vi "Prog11.vi"() -> ()   [LabVIEW 2021]
panel:
  out "length 7":i32
  out "length 6":i32
  out "length 5":i32
  out "length 3":i32
  out "length 2":i32
  out "length":i32
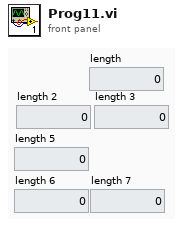
[diagram p1: front panel]
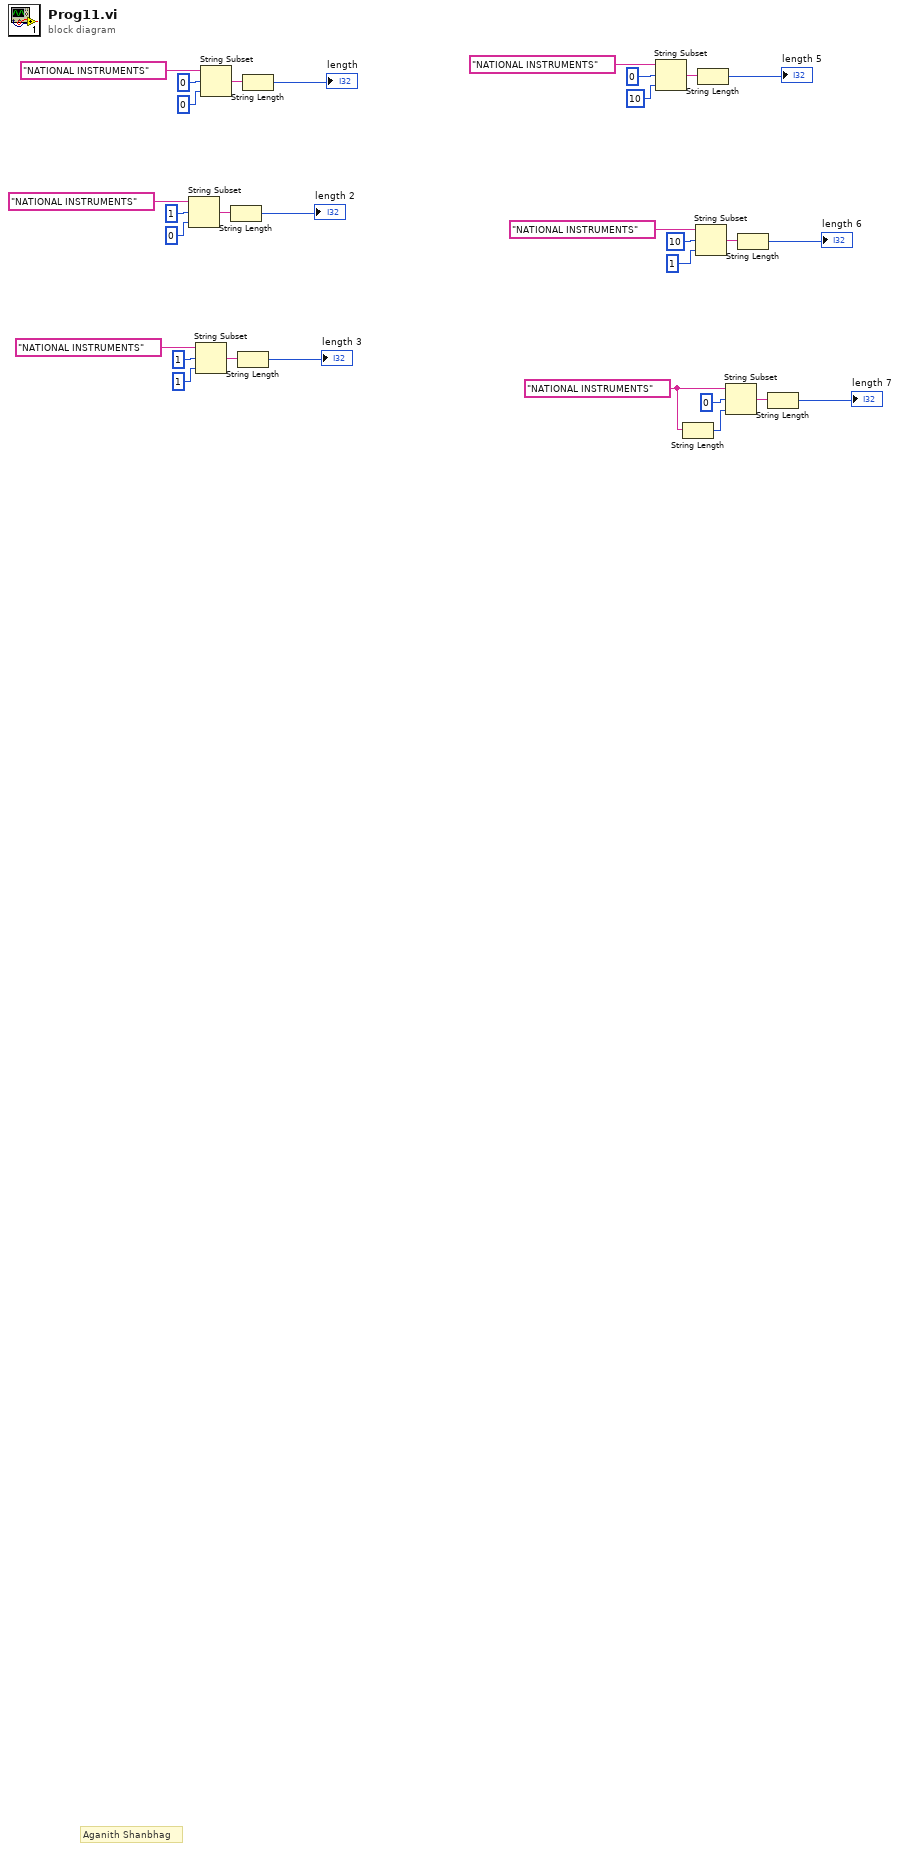
[diagram p0: block diagram]
diagram:
  w10 = "NATIONAL INSTRUMENTS"
  # "Aganith Shanbhag"
  n1 = String Subset(string="NATIONAL INSTRUMENTS", offset (0)=1, length (rest)=0 ("length (rest)")) -> (substring=w21:string)
  n2 = String Subset(string="NATIONAL INSTRUMENTS", offset (0)=1, length (rest)=1 ("length (rest)")) -> (substring=w8:string)
  n3 = String Subset(string="NATIONAL INSTRUMENTS", offset (0)=0, length (rest)=0 ("length (rest)")) -> (substring=w23:string)
  n4 = String Length(string=w21) -> (length=→"length 2":i32)
  n5 = String Length(string=w8) -> (length=→"length 3":i32)
  n6 = String Length(string=w23) -> (length=→"length":i32)
  n7 = String Subset(string="NATIONAL INSTRUMENTS", offset (0)=0, length (rest)=10 ("length (rest)")) -> (substring=w6:string)
  n8 = String Length(string=w10) -> (length=w9:i32)
  n9 = String Subset(string="NATIONAL INSTRUMENTS", offset (0)=10, length (rest)=1 ("length (rest)")) -> (substring=w4:string)
  n10 = String Length(string=w6) -> (length=→"length 5":i32)
  n11 = String Subset(string=w10, offset (0)=0, length (rest)=w9) -> (substring=w2:string)
  n12 = String Length(string=w4) -> (length=→"length 6":i32)
  n13 = String Length(string=w2) -> (length=→"length 7":i32)
